vi "Apply Texture.vi"   [LabVIEW 2017, in "NI_3D Picture Control.lvlib"]
doc: "Maps a texture to the surface of a 3D object. You must manually select the polymorphic instance to use."
uses:
  <vilib>/picture/3D Picture Control/NI_3D Picture Control.lvlib
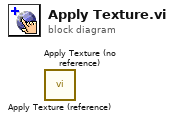
[diagram p0: block diagram]
diagram:
  n1 = call <vilib>:"Apply Texture (reference).vi"() -> ()  [unwired: 9 in, 3 out]
  n2 = call <vilib>:"Apply Texture (no reference).vi"() -> ()  [unwired: 10 in, 2 out]
